vi "Trigger Status Bar.vi"() -> ()   [LabVIEW 2014]
panel:
  out "Trigger Status Bar":bool
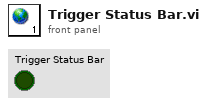
[diagram p1: front panel]
diagram:
